vi "teste-comm.vi"() -> ()   [LabVIEW 2014]
panel:
  out "pfPosition":sgl
  in  "stop":bool
  out "Motor Y\nLigado":bool=TRUE
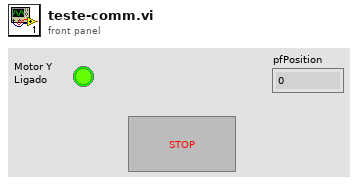
[diagram p1: front panel]
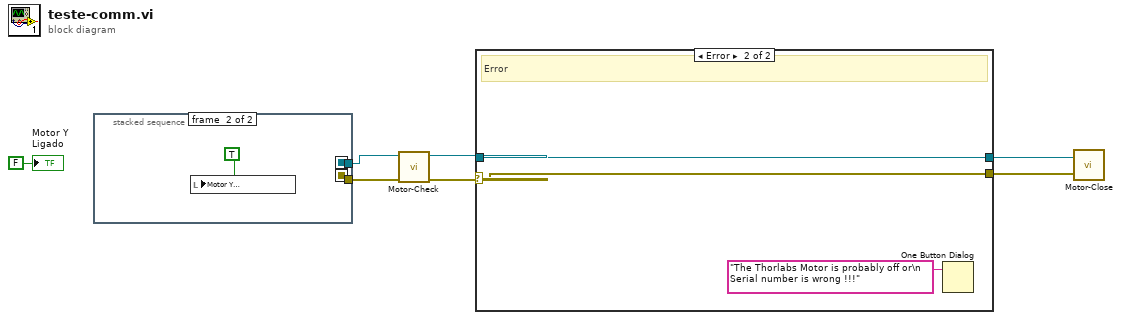
[diagram p0: block diagram]
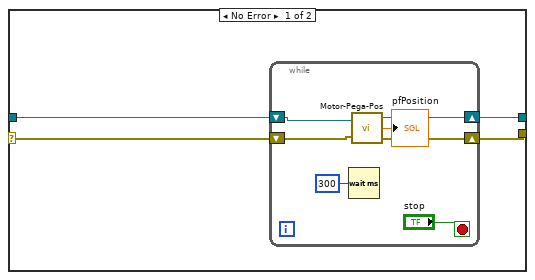
[diagram p2: hidden frame]
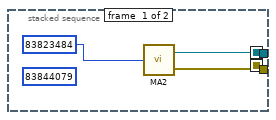
[diagram p3: hidden frame]
diagram:
  n1 = stacked-sequence {
    seq-local: [w10 _] -> [_ w13]
    seq-local: [w9 _] -> [_ w12]
    tunnel: [_ w13] -> w4
    tunnel: [_ w12] -> w2
    frame #0 {
      (unwired) 83844079 ("HWSerialNum")
      n2 = call "MA2.vi"("HWSerialNum"=83823484) -> ("MG17Motor 2"=w10:refnum<k7>, "error out"=w9:errorcluster)
    }
    frame #1 {
      n3 = local write "Motor Y\nLigado"(TRUE ("Motor3\nLigado")) -> ()
    }
  }
  n4 = call "Motor-Check.vi"("error in (no error)"=w2, "Automation Refnum in"=w4) -> ("error out"=w3:errorcluster, "Automation Refnum out"=w1:refnum<k7>)  [unwired: 8 in]
  n5 = case shown="Error" w3 {
    selector: w3 -> [w15 w25]
    tunnel: w1 -> [w14 w26]
    tunnel: [w17 w26] -> w6
    tunnel: [w16 w25] -> w5
    frame No Error {
      n6 = while {
        shift-right: [w22] -> w17
        shift-left: w14 -> [w24]
        shift-right: [w21] -> w16
        shift-left: w15 -> [w23]
        stop <- "stop" stop-if-true
        n7 = Wait (ms)(milliseconds to wait=u32 300) -> ()  [unwired: 1 out]
        n8 = call "Motor-Pega-Pos.vi"("MG17Motor 2"=w24, "error out"=w23) -> ("MG17Motor 3"=w22:refnum<k7>, "pfPosition"=→"pfPosition":sgl, "error out 2"=w21:errorcluster)
      }
    }
    frame Error {
      # "Error"
      n9 = One Button Dialog(message="The Thorlabs Motor is probably off or\n Serial number is wrong !!!") -> ()  [unwired: 1 in, 1 out]
    }
  }
  n10 = call "Motor-Close.vi"("error out"=w5, "MG17Motor 3"=w6) -> ()  [unwired: 1 in]
  "Motor Y\nLigado" <- FALSE ("Motor Y\nLigado")
